vi "EMA(Obj_Det_Train_Stats).vi"(9 "Exp_Avg":sgl, 11 "Det_Train_Stats":T2 {"Loss" format="%.5f"; "Count" format="%.5f"; "Avg_NoObj" format="%.5f"; "Avg_IOU" format="%.5f"; "Avg_Obj" format="%.5f"; "Avg_Class" format="%.5f"; "Avg_Recall" format="%.5f"}) -> (3 "Cluster":T1)   [LabVIEW 2020]
uses:
  <vilib>/Ngene/Deep Learning Toolkit/Toolkit/NN_Loss/API/Controls/NN_Loss_Stats(YOLO_v2).ctl
  <vilib>/Ngene/Deep Learning Toolkit/Toolkit/Deep_Learning_Toolkit_by_Ngene.lvlib
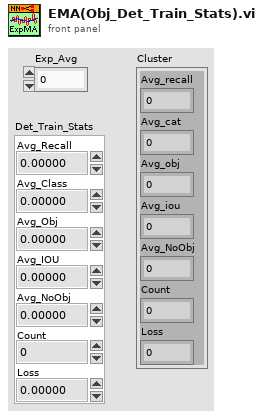
[diagram p1: front panel]
types:
  T1 = cluster{"Avg_recall":sgl, "Avg_cat":sgl, "Avg_obj":sgl, "Avg_iou":sgl, "Avg_NoObj":sgl, "Count":sgl, "Loss":sgl}
  T2 = typedef "Deep_Learning_Toolkit_by_Ngene.lvlib/NN_Loss_Stats(YOLO_v2).ctl" = cluster{"Avg_Recall":sgl, "Avg_Class":sgl, "Avg_Obj":sgl, "Avg_IOU":sgl, "Avg_NoObj":sgl, "Count":i32, "Loss":sgl}
  T3 = cluster{"Avg_Recall":sgl, "Avg_Class":sgl, "Avg_Obj":sgl, "Avg_IOU":sgl, "Avg_NoObj":sgl, "Count":sgl, "Loss":sgl}
  T4 = cluster{sgl, sgl, sgl, sgl, "Avg_NoObj":sgl, "Count":sgl, "Loss":sgl}
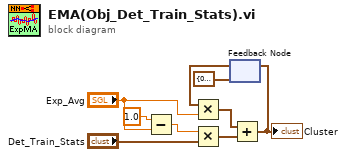
[diagram p0: block diagram]
diagram:
  n1 = Subtract(x=sgl 1.0 ("y"), y="Exp_Avg") -> (x-y=w7:sgl)
  n2 = Multiply(x=w7, y="Det_Train_Stats") -> (x*y=w2:T3)
  n3 = feedback #1(T1 {"Avg_recall"=0.0, "Avg_cat"=0.0, "Avg_obj"=0.0, "Avg_iou"=0.0, "Avg_NoObj"=0.0, "Count"=0.0, "Loss"=0.0}) -> (w4:T1)
  n4 = Multiply(x=w4, y="Exp_Avg") -> (x*y=w5:T1)
  n5 = Add(x=w5, y=w2) -> (x+y=w3:T4)
  "Cluster" <- w3
  n6 = feedback-in #1(w3) -> ()
